vi "ContinuousPressureAcquisition.vi"(8 "error in":errorcluster) -> (0 "error out":errorcluster)   [LabVIEW 2012]
uses:
  GlobalVariables/IndexCaptor.vi
  GlobalVariables/IndexFlowmeter.vi
  GlobalVariables/Samples.vi
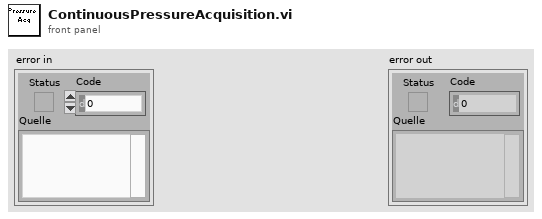
[diagram p1: front panel]
types:
  T1 = cluster{"Pressure":cluster{"TimeSamples":dbl[], "PressureSamples":dbl[]}, "Flow":cluster{"TimeSamples":dbl[], "FlowSamples":dbl[]}}
  T2 = cluster{"TimeSamples":dbl[], "PressureSamples":dbl[]}
  T3 = cluster{"TimeSamples":dbl[], "FlowSamples":dbl[]}
  T4 = cluster{"Values":cluster{dbl[], dbl[]}, "Values":cluster{dbl[], dbl[]}}
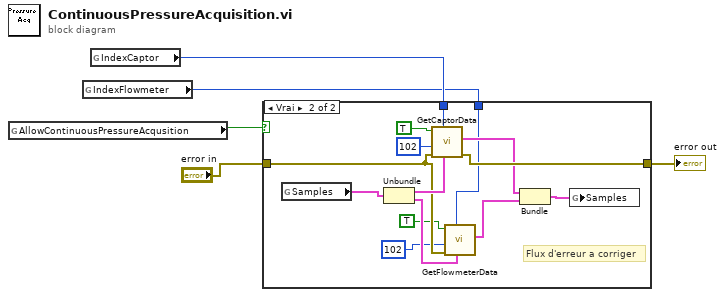
[diagram p0: block diagram]
diagram:
  n1 = global read "AllowContinuousPressureAcquisition.vi" "AllowContinuousPressureAcqusition"() -> (w5:bool)
  n2 = global read "IndexFlowmeter.vi" "IndexFlowmeter"() -> (w1:i32)
  n3 = global read "IndexCaptor.vi" "IndexCaptor"() -> (w2:i32)
  n4 = case shown="Vrai" w5 {
    tunnel: "error in" -> [w6 w11]
    tunnel: [w6 w18] -> w3
    tunnel: w2 -> [_ w8]
    tunnel: w1 -> [_ w7]
    frame False {
    }
    frame True {
      # "Flux d'erreur a corriger"
      n5 = global read "Samples.vi" "Samples"() -> (w16:T1)
      n6 = Unbundle(w16) -> ("Pressure"=w17:T2, "Flow"=w13:T3)
      n7 = call "GetCaptorData.vi"("Graph in"=w17, "Index"=w8, "error in"=w11, "Length"=102, "ON"=TRUE) -> ("error out"=w18:errorcluster, "Values"=w14:cluster{dbl[], dbl[]})  [unwired: 5 in]
      n8 = call "GetFlowmeterData.vi"("Graph in"=w13, "Index"=w7, "error in"=w11, "Length"=102, "ON"=TRUE) -> ("Values"=w12:cluster{dbl[], dbl[]})  [unwired: 5 in, 1 out]
      n9 = Bundle("Values"=w14, "Values"=w12) -> (w15:T4)  [unwired: 1 in]
      n10 = global write "Samples.vi" "Samples"(w15) -> ()
    }
  }
  "error out" <- w3
